vi "Dashboard Main.vi"() -> ()   [LabVIEW 2017]
uses:
  <vilib>/Utility/miscctls.llb/LVRowAndColumnTypeDef.ctl
  <vilib>/event_ctls.llb/eventvkey.ctl
  <vilib>/Rock Robotics/Network Tables/NT Read Numeric Array.vi
  <vilib>/Rock Robotics/Network Tables/NT Write Boolean.vi
  <vilib>/Rock Robotics/WPI/Dashboard/WPI_DashboardLogging Global.vi
panel:
  in  "TCP":refnum<k5>
  in  "Rec Mode":enum32{"Stop", "Record", "Playback"}(radio)
  out "Robot IP":string
  out "Image Message":string="Timeout in Camera Communications"
  in  "Dashboard Tab":T1(tab)
  in  "Drive Type":string(combo)
  in  "ResetGyro":bool
  in  "ResetSwerves":bool
  in  "Select Auto":string(combo)="Select Autonomous ..."
  out "NT Connection":bool
  out "MotorChart R":cluster{"Numeric":dbl, "Numeric":dbl}(graph)
  out "MotorChart L":cluster{"Numeric":dbl, "Numeric":dbl}(graph)
  out "MotorSliders R":cluster{"MotorSlide1":dbl, "MotorSlide2":dbl} {"MotorSlide2" scale=-1.0..1.0 scale format="%#_2e"; "MotorSlide1" scale=-1.0..1.0 scale format="%#_2e"}
  out "MotorSliders L":cluster{"MotorSlide1":dbl, "MotorSlide2":dbl} {"MotorSlide2" scale=-1.0..1.0 scale format="%#_2e"; "MotorSlide1" scale=-1.0..1.0 scale format="%#_2e"}
  out "Gyro":dbl(knob) scale=0.0..360.0
  out "JS1 Z":dbl(slide) scale=-1.0..1.0 scale format="%#_2e"
  out "JS1 Graph":cluster{"X":dbl, "Y":dbl}[](graph)
  out "JS1 Buttons":T2
  out "JS2 Z":dbl(slide) scale=-1.0..1.0 scale format="%#_2e"
  out "JS2 Graph":cluster{"X":dbl, "Y":dbl}[](graph)
  out "JS2 Buttons":T2
  out "Mode":T3(ring)=enum."Auto Disabled"
  in  "DB/String 9":string
  in  "DB/String 8":string
  in  "DB/String 7":string
  in  "DB/String 6":string
  in  "DB/String 5":string
  in  "DB/String 4":string
  in  "DB/String 3":string
  in  "DB/String 2":string
  in  "DB/String 1":string
  in  "DB/String 0":string
  in  "DB/Slider 0":dbl(slide) scale=0.0..5.0
  in  "DB/Slider 1":dbl(slide) scale=0.0..5.0
  in  "DB/Slider 2":dbl(slide) scale=0.0..5.0
  in  "DB/Slider 3":dbl(slide) scale=0.0..5.0
  out "DB/LED 3":bool
  out "DB/LED 2":bool
  out "DB/LED 1":bool
  out "DB/LED 0":bool
  in  "DB/Button 3":bool
  in  "DB/Button 2":bool
  in  "DB/Button 1":bool
  in  "DB/Button 0":bool caption="New Name"
  in  "Test Slider":dbl(slide) scale=0.0..100.0 scale format="%#_3g"
  in  "On/Off":bool caption="Solenoid"
  in  "Test Name":u16(ring) items=["Select the test to run..."]
  in  "Test Tree":string(tree)
  in  "Motor":cluster{"Value":dbl, "Enable":bool} {"Value" scale=-1.0..1.0 scale format="%#_3g"}
  out "Progress":T4 {"Test Progress" scale=0.0..100.0}
  in  "Rev/Fwd":cluster{"Forward":bool, "Reverse":bool}
  in  "Test Ring":u16(ring) items=["Monochrome", "Color"]
  out "Cmd Status":string
  in  "Execute Command":bool
  in  "Command Params":string[][](table)
  in  "Command Selection":i32(listbox)
  in  "CheckList":i32(listbox)
  out "Tree":string(tree)
  out "Background":bool
  # "Joysticks"
  # "Drive Motors"
  # "Front"
  # "Right"
  # "Left"
  # "Back"
  # "This tab is a great place for autonomous settings and robot-specific values.\nPlace controls and indicators inside this tab and match name to\nDashboard Variables on robot. You can also delete this comment."
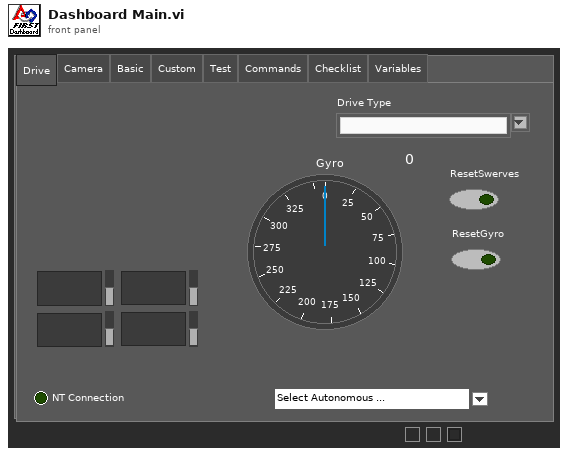
[diagram p1: front panel]
types:
  T1 = enum32{"Drive", "Camera", "Basic", "Custom", "Test", "Commands", "Checklist", "Variables"}
  T2 = cluster{bool, bool, bool, bool, bool, bool, bool, bool, bool, bool, bool, bool}
  T3 = enum8{"Tele-Op Disabled", "Tele-Op Enabled", "Auto Disabled", "Auto Enabled", "Test Disabled", "Test Enabled", "Disconnected", "No Code", "E-Stop"}
  T4 = cluster{"Test Progress":u8, "Test Progress Text":string}
  T5 = cluster{"IDs":cluster{"RPC field ID":u16, "Unique ID":u16}, "String":string}
  T6 = cluster{"Error Strings":string, "Disable Counts":cluster{u16, u16}, "Rail Faults":cluster{u16, u16, u16}, "Robot IP":string, "DB Mode":u8, "Event Info":cluster{"Name":string, "Type":u8, "Number":u16, "Replay":u8}}
  T7 = cluster{"Storage":cluster{"Disk Free":u64, "RAM Block":u32, "RAM free":u32}, "CPU Utilization":cluster{"CPU % ISR":sgl, "CPU % Time Crit":sgl, "CPU % Timed Str":sgl, "CPU % High":sgl, "CPU % Above":sgl, "CPU % Normal":sgl, "CPU % Low":sgl}, "CAN":cluster{"% Bus Utilization":sgl, "Bus Off Cnt":u32, "TX_FIFO Full Cnt":u32, "Receive Error Cnt":u8, "Transmit Error Cnt":u8}, "HID":cluster{"HID Outputs":u32, "Rumble Low":u16, "Rumble High":u16}[]}
  T8 = cluster{"Status bits":cluster{"Test Mode":bool, "Autonomous":bool, "Enabled":bool, "Code Start":bool, "Brownout":bool, "Reserved 2":bool, "Reserved 3":bool, "E-Stop":bool}, "Code Trace":cluster{"Disabled":bool, "TeleOp":bool, "Auto":bool, "Test":bool}, "Controller Type":enum16{"unknown", "cRIO", "roboRio"}, "Code?":enum16{"unknown", "noCode", "code"}, "Battery V":dbl}
  T9 = cluster{"Control Bits":cluster{"TestMode":bool, "Autonomous":bool, "Enabled":bool, "FMS Present":bool, bool, bool, bool, "E-Stop":bool}, "Team Station ":u8, "Countdown":sgl, "Joystick Values":cluster{"Axes":dbl[], "Buttons":bool[], "POVs":i16[]}[]}
  T10 = cluster{"Axes":dbl[], "Buttons":bool[], "POVs":i16[]}[]
  T11 = cluster{"Axes":dbl[], "Buttons":bool[], "POVs":i16[]}
  T12 = cluster{"Buttons[0]":bool, "Buttons[1]":bool, "Buttons[2]":bool, "Buttons[3]":bool, "Buttons[4]":bool, "Buttons[5]":bool, "Buttons[6]":bool, "Buttons[7]":bool, "Buttons[8]":bool, "Buttons[9]":bool, "Buttons[10]":bool, "Buttons[11]":bool}
  T13 = cluster{"Operation":enum16{"Update", "Clear"}, "Color Box":u32}[]
  T14 = typedef "eventvkey.ctl" = enum16{"ASCII", "Enter", "Return", "Shift", "Ctrl", "Alt", "Cmd", "Opt", "Caps", "NumLock", "Clear", "Break", "Up", "Down", "Left", "Right", "Insert", "Delete", "Home", "End", "PageUp", "PageDown", "Escape", "Help", "Pause", "ScrollLock", "F1", "F2", "F3", "F4", "F5", "F6", "F7", "F8", "F9", "F10", "F11", "F12", "F13", "F14", "F15", "F16", "F17", "F18", "F19", "F20", "F21", "F22", "F23", "F24", "Play", "VolumeUp", "VolumeDown", "Mute", "Two Byte Char"}
  T15 = cluster{"Image Size":bool, "Image Type":bool, "Pixel Value":bool, "ROI Information":bool, "Zoom Factor":bool}
  T16 = cluster{"Operation":enum16{"Update", "Clear"}, "Color Box":u32}
  T17 = typedef "LVRowAndColumnTypeDef.ctl" = cluster{"Row":i32, "Column":i32}
  T18 = cluster{"Shift":bool, "Ctrl":bool, "Alt":bool, "Cmd":bool, "Opt":bool}
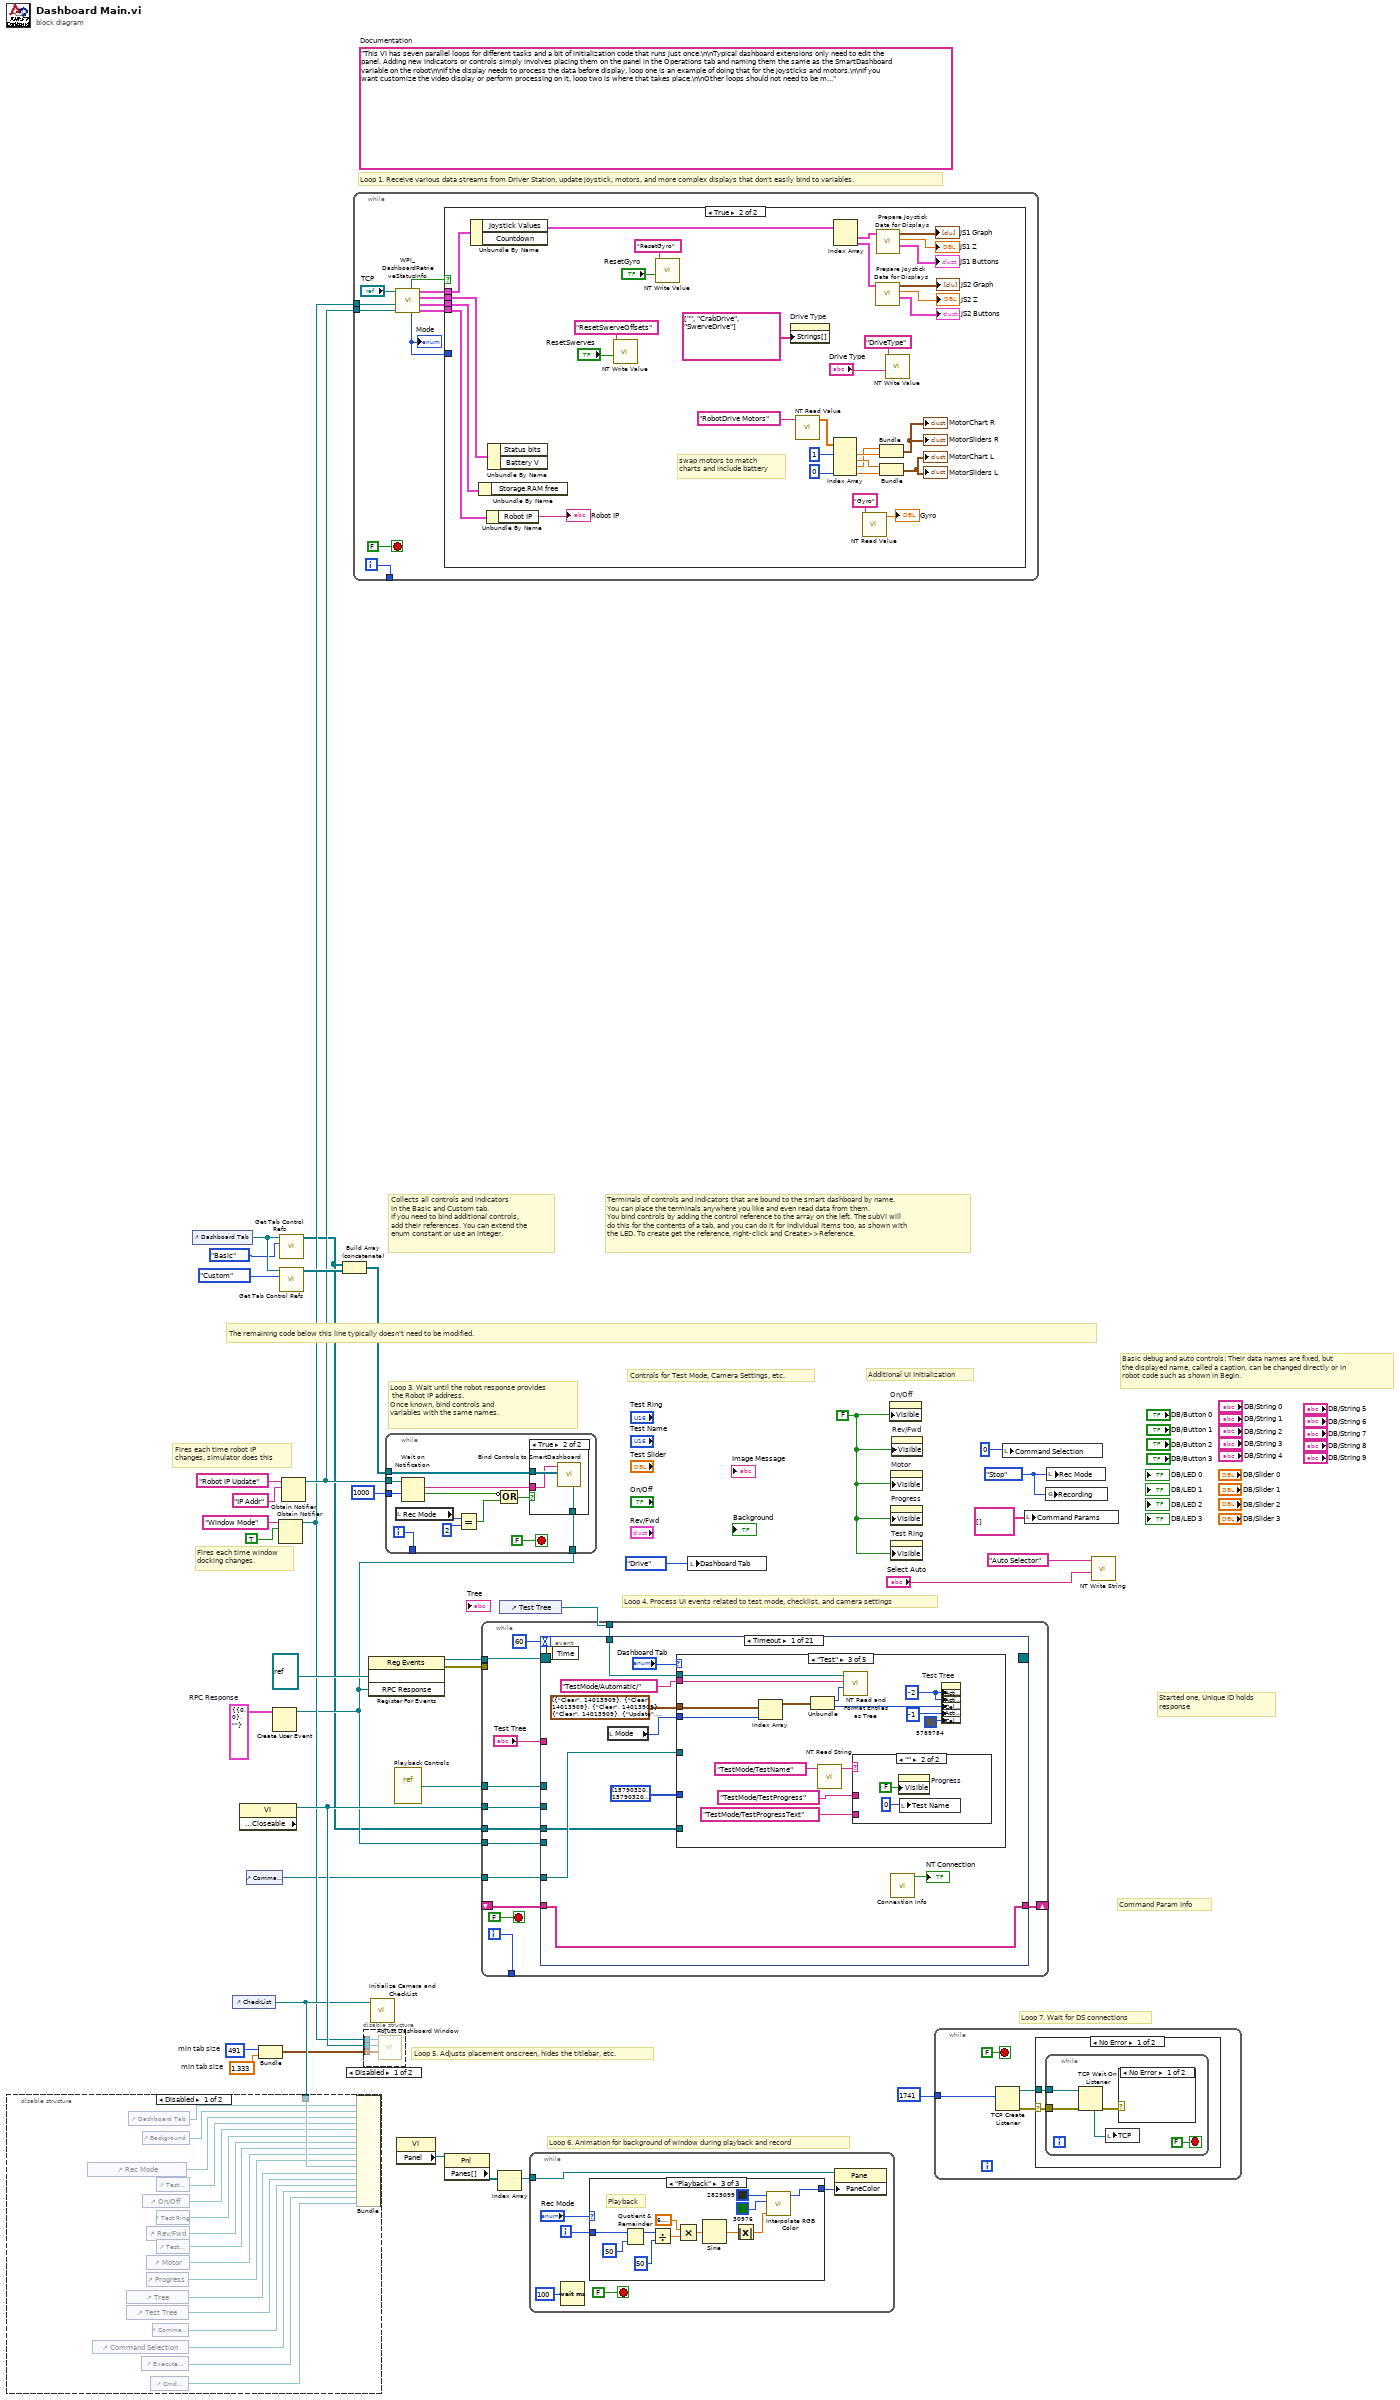
[diagram p0: block diagram]
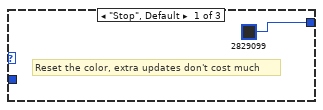
[diagram p4: hidden frame]
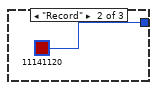
[diagram p5: hidden frame]
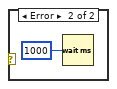
[diagram p6: hidden frame]
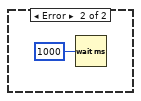
[diagram p7: hidden frame]
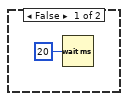
[diagram p8: hidden frame]
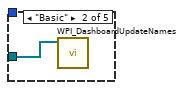
[diagram p11: hidden frame]
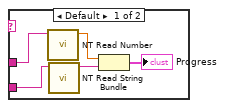
[diagram p12: hidden frame]
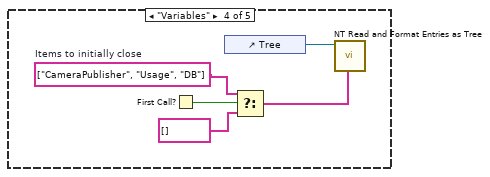
[diagram p13: hidden frame]
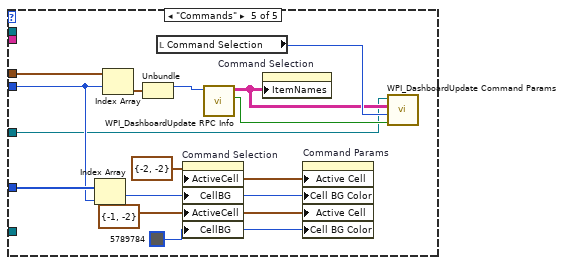
[diagram p14: hidden frame]
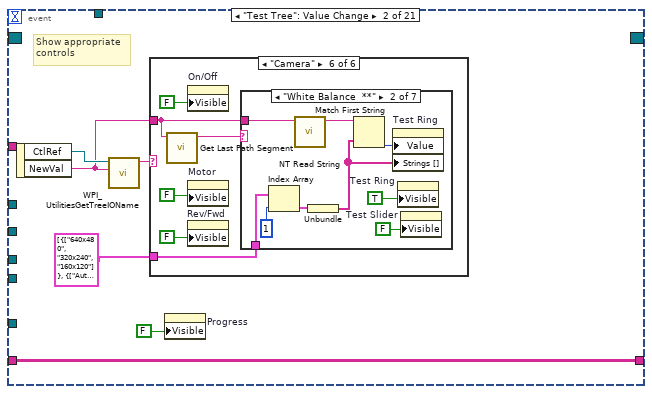
[diagram p15: hidden frame]
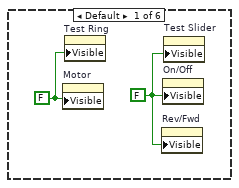
[diagram p16: hidden frame]
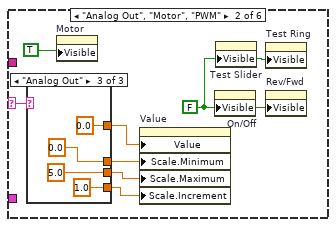
[diagram p17: hidden frame]
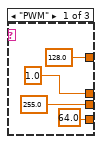
[diagram p18: hidden frame]
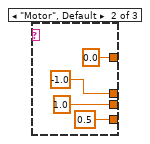
[diagram p19: hidden frame]
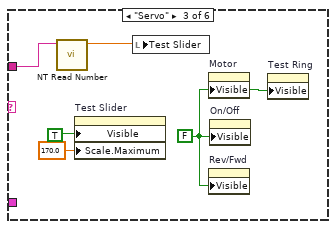
[diagram p20: hidden frame]
diagram:
  w3 = 491  # min tab size
  w2 = 1.333  # min tab size
  w16 = T5 {"IDs"={"RPC field ID"=0, "Unique ID"=0}, "String"=""}  # RPC Response
  w27 = enum32{"Stop", "Record", "Playback"}."Stop" ("Rec Mode")
  w21 = FALSE ("Visible")
  (unwired) "This VI has seven parallel loops for different tasks and a bit of initialization code that runs just once.\n\nTypical dashboard extensions only need to edit the panel. Adding new indicators or controls simply involves placing them on the panel in the Operations tab and naming them the same as the SmartDashboard variable on the robot\n\nIf the display needs to process the data before display, loop one is an example of doing that for the joysticks and motors.\n\nIf you want customize the video display or perform processing on it, loop two is where that takes place.\n\nOther loops should not need to be modified. They are pretty standard, and document the task they perform."  # Documentation
  # "Loop 5. Adjusts placement onscreen, hides the titlebar, etc."
  # "Loop 6. Animation for background of window during playback and record"
  # "Command Param Info"
  # "Started one, Unique ID holds\nresponse"
  # "Loop 7. Wait for DS connections"
  # "Basic debug and auto controls: Their data names are fixed, but\nthe displayed name, called a caption, can be changed directly or in\nrobot code such as shown in Begin."
  # "Controls for Test Mode, Camera Settings, etc."
  # "Additional UI Initialization"
  # "Fires each time robot IP\nchanges, simulator does this"
  # "Fires each time window\ndocking changes."
  # "Collects all controls and indicators\nin the Basic and Custom tab.\nIf you need to bind additional controls,\nadd their references. You can extend the\nenum constant or use an integer."
  # "The remaining code below this line typically doesn't need to be modified."
  # "Loop 4. Process UI events related to test mode, checklist, and camera settings"
  # "Terminals of controls and indicators that are bound to the smart dashboard by name.\nYou can place the terminals anywhere you like and even read data from them.\nYou bind controls by adding the control reference to the array on the left. The subVI will\ndo this for the contents of a tab, and you can do it for individual items too, as shown with\nthe LED. To create get the reference, right-click and Create>>Reference."
  # "Loop 3. Wait until the robot response provides\n the Robot IP address.\nOnce known, bind controls and\nvariables with the same names."
  # "Loop 1. Receive various data streams from Driver Station, update joystick, motors, and more complex displays that don't easily bind to variables."
  n1 = control-ref of="Dashboard Tab"() -> (w25:refnum<vi>)
  n2 = control-ref of="CheckList"() -> (w22:refnum<vi>)
  n3 = disable-structure shown="Disabled" {
    disable-tunnel: w22 -> [w54 _]
    frame Disabled {
      n4 = control-ref of="Rec Mode"() -> (w47:refnum<vi>)
      n5 = control-ref of="Command Selection"() -> (w39:refnum<vi>)
      n6 = control-ref of="Tree"() -> (w51:refnum<vi>)
      n7 = control-ref of="Test Tree"() -> (w50:refnum<vi>)
      n8 = control-ref of="Dashboard Tab"() -> (w53:refnum<vi>)
      n9 = control-ref of="Execute Command"() -> (w40:refnum<vi>)
      n10 = control-ref of="Background"() -> (w52:refnum<vi>)
      n11 = control-ref of="On/Off"() -> (w45:refnum<vi>)
      n12 = control-ref of="Progress"() -> (w42:refnum<vi>)
      n13 = control-ref of="Rev/Fwd"() -> (w43:refnum<vi>)
      n14 = control-ref of="Motor"() -> (w48:refnum<vi>)
      n15 = control-ref of="Cmd Status"() -> (w38:refnum<vi>)
      n16 = control-ref of="Command Params"() -> (w41:refnum<vi>)
      n17 = control-ref of="Test Slider"() -> (w46:refnum<vi>)
      n18 = control-ref of="Test Ring"() -> (w44:refnum<vi>)
      n19 = control-ref of="Test Name"() -> (w49:refnum<vi>)
      n20 = Bundle("Dashboard Tab"=w53, "Background"=w52, "Rec Mode"=w47, "Test Slider"=w46, "On/Off"=w45, "Test Ring"=w44, "Rev/Fwd"=w43, "Test Name"=w49, "Motor"=w48, "Progress"=w42, "CheckList"=w54, "Tree"=w51, "Test Tree"=w50, "Command Params"=w41, "Command Selection"=w39, "Execute Command"=w40, "Cmd Status"=w38) -> ()  [unwired: 2 in, 1 out]
    }
    frame Enabled {
    }
  }
  n21 = property class="VI" props=["Front Panel.Closeable"]() -> (reference out=w26:refnum<vi>)  [unwired: 2 in, 2 out]
  n22 = control-ref of="Command Params"() -> (w12:refnum<vi>)
  n23 = Bundle("min tab size"=w3, "min tab size"=w2) -> (w1:cluster{"min tab size":i32, "min tab size":dbl})  [unwired: 1 in]
  n24 = Create User Event(user event datatype=w16) -> (user event=w13:refnum<user-event>)  [unwired: 1 in, 1 out]
  n25 = Obtain Notifier(name (unnamed)="Window Mode", notification data type=TRUE) -> (notifier out=w19:refnum<notifier>)  [unwired: 2 in, 2 out]
  n26 = call <vilib>:"Get Tab Control Refs.vi"("Page Index"=T1."Basic" ("Dashboard Tab"), "TabControl in"=w25) -> ("ControlsOnPage"=w11:refnum<vi>[])  [unwired: 9 in]
  n27 = call <vilib>:"Get Tab Control Refs.vi"("Page Index"=T1."Custom" ("Dashboard Tab"), "TabControl in"=w25) -> ("ControlsOnPage"=w24:refnum<vi>[])  [unwired: 9 in]
  n28 = Obtain Notifier(name (unnamed)="Robot IP Update", notification data type="IP Addr" ("name (unnamed)")) -> (notifier out=w20:refnum<notifier>)  [unwired: 2 in, 2 out]
  n29 = Build Array (concatenate)(w11, w24) -> (w23:refnum<vi>[])
  n30 = while {
    tunnel: [w64] -> _
    tunnel: w20 -> [w58]
    tunnel: w19 -> [w55]
    i -> [w64]
    stop <- FALSE stop-if-true
    n31 = call <vilib>:"WPI_DashboardRetrieveStatusInfo.vi"("Binding Refnum"=w58, "Window Mode Notifier"=w55, "TCP Cnx"="TCP") -> ("Power and Errors"=w59:T6, "Robot Metrics"=w62:T7, "Status Info"=w63:T8, "Control Info"=w60:T9, "Robot Mode"=w57:T3, "Process?"=w61:bool)  [unwired: 3 in]
    "Mode" <- w57
    n32 = case shown="True" w61 {
      tunnel: w63 -> [_ w99]
      tunnel: w62 -> [_ w98]
      tunnel: w60 -> [_ w97]
      tunnel: w59 -> [_ w96]
      tunnel: w57 -> [_ _]
      frame False {
        n33 = Wait (ms)(milliseconds to wait=u32 20) -> ()  [unwired: 1 out]
      }
      frame True {
        # "swap motors to match\ncharts and include battery"
        n34 = Unbundle By Name(w97) -> ("Joystick Values"=w87:T10)  [unwired: 1 out]
        n35 = Unbundle By Name(w98) -> ()  [unwired: 1 out]
        n36 = Unbundle By Name(w96) -> ("Robot IP"=→"Robot IP":string)
        n37 = Unbundle By Name(w99) -> ()  [unwired: 2 out]
        n38 = call-poly <vilib>:"NT Write Value.vi"("Boolean"="ResetSwerves", "Name"="ResetSwerveOffsets") -> ()  [unwired: 9 in, 1 out]
        n39 = call-poly <vilib>:"NT Write Value.vi"("Boolean"="ResetGyro", "Name"="ResetGyro") -> ()  [unwired: 9 in, 1 out]
        n40 = property on="Drive Type" class="CmbBox"("Strings[]"=string[] ["", "CrabDrive", "SwerveDrive"] ("Strings []")) -> ()  [unwired: 2 in, 2 out]
        n41 = call-poly <vilib>:"NT Read Value.vi"("Name"="RobotDrive Motors") -> ("Numeric Array"=w77:dbl[])  [unwired: 9 in, 1 out]
        n42 = Index Array(array=w77, index #1=1, index #4=0) -> (element #1=w91:dbl, element #2=w92:dbl, element #3=w90:dbl, element #4=w95:dbl)  [unwired: 2 in]
        n43 = Index Array(array=w87) -> (element #1=w86:T11, element #2=w82:T11)  [unwired: 2 in]
        n44 = call-poly <vilib>:"NT Read Value.vi"("Name"="Gyro") -> ("Numeric"=→"Gyro":dbl)  [unwired: 9 in, 1 out]
        n45 = call "Prepare Joystick Data for Displays.vi"("Joystick Values"=w82) -> ("Buttons"=→"JS2 Buttons":T12, "Z Axis"=→"JS2 Z":dbl, "Cartesian Data"=→"JS2 Graph":cluster{"X axis":dbl, "X axis":dbl}[])  [unwired: 8 in]
        n46 = call "Prepare Joystick Data for Displays.vi"("Joystick Values"=w86) -> ("Buttons"=→"JS1 Buttons":T12, "Z Axis"=→"JS1 Z":dbl, "Cartesian Data"=→"JS1 Graph":cluster{"X axis":dbl, "X axis":dbl}[])  [unwired: 8 in]
        n47 = Bundle("Numeric"=w90, "Numeric"=w91) -> (→"MotorChart R" →"MotorSliders R":cluster{"Numeric":dbl, "Numeric":dbl})  [unwired: 1 in]
        n48 = Bundle("Numeric"=w92, "Numeric"=w95) -> (→"MotorChart L" →"MotorSliders L":cluster{"Numeric":dbl, "Numeric":dbl})  [unwired: 1 in]
        n49 = call-poly <vilib>:"NT Write Value.vi"("String"="Drive Type", "Name"="DriveType") -> ()  [unwired: 9 in, 1 out]
      }
    }
  }
  n50 = disable-structure shown="Disabled" {
    disable-tunnel: w26 -> [w102 _]
    disable-tunnel: w19 -> [w101 _]
    disable-tunnel: w1 -> [w100 _]
    frame Disabled {
      n51 = call "Adjust Dashboard Window.vi"("Size Constraints"=w100, "VI"=w102, "WIn Mode"=w101) -> ()  [unwired: 9 in]
    }
    frame Enabled {
    }
  }
  n52 = register-events(refnum<vi> refnum, w13) -> (reference out=w31:refnum<event-registration>, error out=w30:errorcluster)  [unwired: 2 in]
  n53 = call "Initialize Camera and CheckList.vi"("ListBox in"=w22) -> ()  [unwired: 11 in]
  n54 = while {
    tunnel: w23 -> [w114]
    tunnel: w20 -> [w112]
    tunnel: [w110] -> _
    tunnel: u32 1000 ("milliseconds to wait") -> [w109]
    tunnel: w13 -> [w103]
    i -> [w110]
    stop <- FALSE stop-if-true
    n55 = local read "Rec Mode"() -> (w105:enum32{"Stop", "Record", "Playback"})
    n56 = Wait on Notification(notifier=w112, timeout in ms (-1)=w109) -> (notification=w111:string, timed out?=w107:bool)  [unwired: 2 in, 2 out]
    n57 = Equal?(x=w105, y=u16 2 ("Rec Mode")) -> (x = y?=w106:bool)
    n58 = Compound Arithmetic op=OR(invert w107, w106) -> (w108:bool)
    n59 = case shown="True" w108 {
      tunnel: w114 -> [_ w117]
      tunnel: w111 -> [_ w116]
      tunnel: w103 -> [_ w115]
      frame False {
      }
      frame True {
        n60 = call <vilib>:"Bind Controls to SmartDashboard.vi"("RPC ref"=w115, "Bound Control Refs"=w117, "Server IP Address"=w116) -> ()  [unwired: 9 in]
      }
    }
  }
  n61 = vi-ref "Playback Controls.vi"() -> (w32:refnum<vi>)
  n62 = property class="VI"() -> ("Panel"=w5:refnum<vi>)  [unwired: 2 in, 2 out]
  n63 = property class="Pnl"(reference=w5) -> ("Panes[]"=w6:refnum<vi>[])  [unwired: 1 in, 2 out]
  n64 = Index Array(array=w6) -> (element=w4:refnum<vi>)  [unwired: 1 in]
  n65 = control-ref of="Test Tree"() -> (w33:refnum<vi>)
  n66 = while {
    tunnel: [w127] -> _
    tunnel: w33 -> [w126]
    tunnel: w32 -> [w125]
    tunnel: w31 -> [w124]
    tunnel: w30 -> [_]
    tunnel: w26 -> [w123]
    tunnel: w13 -> [w122]
    tunnel: w12 -> [w121]
    shift-right: [w120] -> _
    shift-left: _ -> [w119]
    tunnel: w11 -> [w118]
    i -> [w127]
    stop <- FALSE stop-if-true
    n67 = event shown="[0] Timeout" {
      selector: w124 -> [_ _ _ _ _ _ _ _ _ _ _ _ _ _ _ _ _ _ _ _ _]
      dyn-events: [_ _ _ _ _ _ _ _ _ _ _ _ _ _ _ _ w385 _ _ _ _] -> _
      timeout: u32 60 ("milliseconds to wait") -> [_ _ _ _ _ _ _ _ _ _ _ _ _ _ _ _ _ _ _ _ _]
      tunnel: w126 -> [w139 _ _ _ _ _ _ _ _ _ _ _ _ _ _ _ _ _ _ _ _]
      tunnel: "Test Tree" -> [_ _ _ _ _ _ _ _ _ _ _ w354 w362 w364 w368 w376 _ _ _ _ _]
      tunnel: w125 -> [_ _ _ _ _ _ _ _ _ _ _ _ _ _ _ _ w387 _ w405 _ _]
      tunnel: w123 -> [_ _ _ _ _ _ _ _ _ _ _ _ _ _ _ _ w383 _ _ _ _]
      tunnel: w122 -> [_ _ _ _ _ _ _ _ _ _ _ _ _ _ _ _ w381 _ _ _ _]
      tunnel: w121 -> [w134 _ _ _ _ _ w305 _ _ _ _ _ _ _ _ _ _ _ _ _ _]
      tunnel: [w133 w182 w284 w289 w298 w302 w303 w312 w322 w329 w341 w353 w360 w363 w367 w375 w380 w400 w402 w406 w419] -> w120
      tunnel: w119 -> [w133 w182 w284 w289 w298 w302 w303 _ _ w329 w341 w353 w360 w363 w367 w375 w380 w400 w402 w406 w419]
      tunnel: w118 -> [w131 _ _ _ _ _ _ _ _ _ _ _ _ _ _ _ _ _ _ _ _]
      event Timeout {
        n68 = event-data() -> ()  [unwired: 1 in, 1 out]
        n69 = local read "Mode"() -> (w136:T3)
        n70 = case shown="\"Test\"" "Dashboard Tab" {
          tunnel: w139 -> [_ _ w155 _ _]
          tunnel: "TestMode/Automatic/" ("Name Pattern") -> [_ _ w154 _ _]
          tunnel: T13 [{"Operation"=enum."Clear", "Color Box"=14013909}, {"Operation"=enum."Clear", "Color Box"=14013909}, {"Operation"=enum."Clear", "Color Box"=14013909}, {"Operation"=enum."Clear", "Color Box"=14013909}, {"Operation"=enum."Update", "Color Box"=14013909}, {"Operation"=enum."Update", "Color Box"=16777215}, {"Operation"=enum."Clear", "Color Box"=14013909}, {"Operation"=enum."Clear", "Color Box"=14013909}, {"Operation"=enum."Clear", "Color Box"=14013909}] -> [_ _ w147 _ w175]
          tunnel: w136 -> [_ _ w146 _ w174]
          tunnel: u32[] [15790320, 15790320, 15790320, 15790320, 16777215, 16777215, 15790320, 15790320, 15790320] -> [_ _ _ _ w180]
          tunnel: w134 -> [_ _ _ _ w168]
          tunnel: w131 -> [_ w141 _ _ _]
          frame "Custom", Default {
          }
          frame "Basic" {
            n71 = call <vilib>:"WPI_DashboardUpdateNames.vi"("Controls on Tab"=w141) -> ()  [unwired: 11 in]
          }
          frame "Test" {
            w153 = -2 ("Active Item:Row Number")
            n72 = Index Array(array=w147, index=w146) -> (element=w148:T16)
            n73 = Unbundle(w148) -> ("Operation"=w149:enum16{"Update", "Clear"}, "Color Box"=w150:u32)
            n74 = call <vilib>:"NT Read String.vi"("Name"="TestMode/TestName") -> ("String"=w144:string)  [unwired: 9 in, 1 out]
            n75 = call <vilib>:"NT Read and Format Entries as Tree.vi"("Operation"=w149, "Name Pattern"=w154, "Tree Refnum"=w155) -> ()  [unwired: 7 in, 2 out]
            n76 = case shown="\"\"" w144 {
              tunnel: "TestMode/TestProgress" ("Name") -> [w157 _]
              tunnel: "TestMode/TestProgressText" ("Name") -> [w156 _]
              frame Default {
                n77 = call <vilib>:"NT Read Number.vi"("Name"=w157) -> ("Numeric"=w158:dbl)  [unwired: 9 in, 1 out]
                n78 = call <vilib>:"NT Read String.vi"("Name"=w156) -> ("String"=w159:string)  [unwired: 9 in, 1 out]
                n79 = Bundle("Numeric"=w158, "String"=w159) -> (→"Progress":cluster{"Numeric":dbl, "String":string})  [unwired: 1 in]
              }
              frame "" {
                n80 = property on="Progress" class="Clust (strict)"("Visible"=FALSE) -> ()  [unwired: 2 in, 2 out]
                n81 = local write "Test Name"(u16 0) -> ()
              }
            }
            n82 = property on="Test Tree" class="Tree (strict)"("Active Item Row Number"=w153, "ActiveColNum"=w153, "CellBG"=w150, "Active Item Row Number"=-1 ("Active Item:Row Number"), "CellBG"=u32 5789784 ("Color Box")) -> ()  [unwired: 2 in, 2 out]
          }
          frame "Variables" {
            w165 = string[] ["CameraPublisher", "Usage", "DB"]  # Items to initially close
            n83 = First Call?() -> (First Call?: T/F=w166:bool)
            n84 = control-ref of="Tree"() -> (w167:refnum<vi>)
            n85 = Select(t=w165, s=w166, f=string[] []) -> (s? t:f=w163:string[])
            n86 = call <vilib>:"NT Read and Format Entries as Tree.vi"("Tags to  Close"=w163, "Tree Refnum"=w167) -> ()  [unwired: 8 in, 2 out]
          }
          frame "Commands" {
            w176 = u32 5789784 ("Color Box")
            w177 = T17 {"Row"=-1, "Column"=-2} ("Active Cell:Active Cell")
            w179 = T17 {"Row"=-2, "Column"=-2} ("Active Cell:Active Cell")
            n87 = Index Array(array=w180, index=w174) -> (element=w178:u32)
            n88 = Index Array(array=w175, index=w174) -> (element=w173:T16)
            n89 = Unbundle(w173) -> ("Operation"=w172:enum16{"Update", "Clear"})  [unwired: 1 out]
            n90 = local read "Command Selection"() -> (w171:i32)
            n91 = property on="Command Selection" class="MCListbox (strict)"("ActiveCell"=w179, "CellBG"=w178, "ActiveCell"=w177, "CellBG"=w176) -> ()  [unwired: 2 in, 2 out]
            n92 = call <vilib>:"WPI_DashboardUpdate RPC Info.vi"("Operation"=w172) -> ("update"=w170:bool, "commands"=w169:string[][])  [unwired: 9 in]
            n93 = property on="Command Selection" class="MCListbox (strict)"("ItemNames"=w169) -> ()  [unwired: 2 in, 2 out]
            n94 = property on="Command Params" class="Tbl (strict)"("Active Cell"=w179, "Cell BG Color"=w178, "Active Cell"=w177, "Cell BG Color"=w176) -> ()  [unwired: 2 in, 2 out]
            n95 = call <vilib>:"WPI_DashboardUpdate Command Params.vi"("Update"=w170, "NewVal"=w171, "Commands"=w169, "Param Tbl"=w168) -> ()  [unwired: 7 in, 1 out]
          }
        }
        n96 = call <vilib>:"Connextion Info.vi"() -> ("Connected"=→"NT Connection":bool)  [unwired: 10 in, 1 out]
      }
      event "Test Tree": Value Change {
        # "Show appropriate\ncontrols"
        n97 = event-data() -> ("CtlRef"=w185:refnum<vi>, "NewVal"=w183:string)  [unwired: 1 in]
        n98 = call <vilib>:"WPI_UtilitiesGetTreeIOName.vi"("NewVal"=w183, "TreeControl in"=w185) -> ("I/O Name"=w186:string)  [unwired: 9 in]
        n99 = case shown="\"Camera\"" w186 {
          selector: w186 -> [_ w193 _ w215 w224 _]
          tunnel: w183 -> [_ _ w212 w214 _ w231]
          tunnel: cluster{string[]}[] [{["640x480", "320x240", "160x120"]}, {["Auto", "Fixed indoor", "Fixed outdoor 1", "Fixed outdoor 2", "Fixed fluorescent 1", "Fixed fluorescent 2", "Hold current"]}, {["Auto", "Flicker-free 50 Hz", "Flicker-free 60 Hz", "Hold current"]}, {["None", "Prioritize frame rate", "Prioritize image quality"]}, {["Monochrome", "Color"]}] -> [_ _ _ _ _ w230]
          frame Default {
            w188 = FALSE ("Visible")
            w187 = FALSE ("Visible")
            n100 = property on="Motor" class="Clust (strict)"("Visible"=w187) -> ()  [unwired: 2 in, 2 out]
            n101 = property on="Test Ring" class="Ring (strict)"("Visible"=w187) -> ()  [unwired: 2 in, 2 out]
            n102 = property on="Rev/Fwd" class="Clust (strict)"("Visible"=w188) -> ()  [unwired: 2 in, 2 out]
            n103 = property on="On/Off" class="Bool (strict)"("Visible"=w188) -> ()  [unwired: 2 in, 2 out]
            n104 = property on="Test Slider" class="Slide (strict)"("Visible"=w188) -> ()  [unwired: 2 in, 2 out]
          }
          frame "Analog Out", "Motor", "PWM" {
            w194 = FALSE ("Visible")
            n105 = case shown="\"Analog Out\"" w193 {
              tunnel: [1.0 ("Value") -1.0 ("Value") 0.0 ("Value")] -> w192
              tunnel: [255.0 ("Value") 1.0 ("Value") 5.0 ("Value")] -> w191
              tunnel: [128.0 ("Value") 0.0 ("Value") 0.0 ("Value")] -> w190
              tunnel: [64.0 ("Value") 0.5 ("Value") 1.0 ("Value")] -> w189
              frame "PWM" {
              }
              frame "Motor", Default {
              }
              frame "Analog Out" {
              }
            }
            n106 = property on="Motor" class="Clust (strict)"("Visible"=TRUE) -> ()  [unwired: 2 in, 2 out]
            n107 = property on="Value" class="Slide (strict)"("Value"=w190, "Scale.Minimum"=w192, "Scale.Maximum"=w191, "Scale.Increment"=w189) -> ()  [unwired: 2 in, 2 out]
            n108 = property on="On/Off" class="Bool (strict)"("Visible"=w194) -> ()  [unwired: 2 in, 2 out]
            n109 = property on="Test Slider" class="Slide (strict)"("Visible"=w194) -> ()  [unwired: 2 in, 2 out]
            n110 = property on="Test Ring" class="Ring (strict)"("Visible"=w194) -> ()  [unwired: 2 in, 2 out]
            n111 = property on="Rev/Fwd" class="Clust (strict)"("Visible"=w194) -> ()  [unwired: 2 in, 2 out]
          }
          frame "Servo" {
            w210 = FALSE ("Visible")
            n112 = call <vilib>:"NT Read Number.vi"("Name"=w212) -> ("Numeric"=w211:dbl)  [unwired: 9 in, 1 out]
            n113 = property on="Test Slider" class="Slide (strict)"("Visible"=TRUE, "Scale.Maximum"=170.0 ("Scale.Range:Maximum")) -> ()  [unwired: 2 in, 2 out]
            n114 = local write "Test Slider"(w211) -> ()
            n115 = property on="Motor" class="Clust (strict)"("Visible"=w210) -> ()  [unwired: 2 in, 2 out]
            n116 = property on="Rev/Fwd" class="Clust (strict)"("Visible"=w210) -> ()  [unwired: 2 in, 2 out]
            n117 = property on="On/Off" class="Bool (strict)"("Visible"=w210) -> ()  [unwired: 2 in, 2 out]
            n118 = property on="Test Ring" class="Ring (strict)"("Visible"=w210) -> ()  [unwired: 2 in, 2 out]
          }
          frame "Relay", "Solenoid" {
            w213 = FALSE ("Visible")
            n119 = property on="Motor" class="Clust (strict)"("Visible"=w213) -> ()  [unwired: 2 in, 2 out]
            n120 = property on="Test Slider" class="Slide (strict)"("Visible"=w213) -> ()  [unwired: 2 in, 2 out]
            n121 = Search and Replace String(input string=w214, search string="/Value  **", replace string="/Direction") -> (result string=w220:string)  [unwired: 5 in, 3 out]
            n122 = property on="Test Ring" class="Ring (strict)"("Visible"=w213) -> ()  [unwired: 2 in, 2 out]
            n123 = call <vilib>:"NT Read String.vi"("Name"=w220) -> ("String"=w218:string)  [unwired: 9 in, 1 out]
            n124 = Equal?(x="Both directions", y=w218) -> (x = y?=w216:bool)
            n125 = Not(x=w216) -> (.not. x?=w217:bool)
            n126 = property on="Rev/Fwd" class="Clust (strict)"("Visible"=w216) -> ()  [unwired: 2 in, 2 out]
            n127 = property on="On/Off" class="Bool (strict)"("Visible"=w217, "Caption.Text"=w215) -> ()  [unwired: 2 in, 2 out]
          }
          frame "Compressor", "Digital Out" {
            w223 = FALSE ("Visible")
            # "Get direction and finish"
            n128 = property on="Motor" class="Clust (strict)"("Visible"=w223) -> ()  [unwired: 2 in, 2 out]
            n129 = property on="Test Slider" class="Slide (strict)"("Visible"=w223) -> ()  [unwired: 2 in, 2 out]
            n130 = property on="Test Ring" class="Ring (strict)"("Visible"=w223) -> ()  [unwired: 2 in, 2 out]
            n131 = property on="On/Off" class="Bool (strict)"("Visible"=TRUE, "Caption.Text"=w224) -> ()  [unwired: 2 in, 2 out]
            n132 = property on="Rev/Fwd" class="Clust (strict)"("Visible"=FALSE) -> ()  [unwired: 2 in, 2 out]
          }
          frame "Camera" {
            n133 = call <vilib>:"Get Last Path Segment.vi"("String in"=w231) -> ("String out"=w232:string)  [unwired: 10 in]
            n134 = property on="On/Off" class="Bool (strict)"("Visible"=FALSE) -> ()  [unwired: 2 in, 2 out]
            n135 = property on="Motor" class="Clust (strict)"("Visible"=FALSE) -> ()  [unwired: 2 in, 2 out]
            n136 = property on="Rev/Fwd" class="Clust (strict)"("Visible"=FALSE) -> ()  [unwired: 2 in, 2 out]
            n137 = case shown="\"White Balance  **\"" w232 {
              tunnel: w231 -> [w238 w247 w256 w265 w274 _ w280]
              tunnel: w230 -> [w236 w244 w253 w262 w271 _ _]
              frame "Size  **" {
                n138 = Index Array(array=w236) -> (element=w235:cluster{string[]})  [unwired: 1 in]
                n139 = call <vilib>:"NT Read String.vi"("Name"=w238) -> ("String"=w237:string)  [unwired: 9 in, 1 out]
                n140 = Unbundle(w235) -> (w233:string[])
                n141 = Match First String(2:w233, 3:w237) -> (0:w234:i32)  [unwired: 1 out]
                n142 = property on="Test Ring" class="Ring (strict)"("Value"=w234, "Strings []"=w233) -> ()  [unwired: 2 in, 2 out]
                n143 = property on="Test Ring" class="Ring (strict)"("Visible"=TRUE) -> ()  [unwired: 2 in, 2 out]
                n144 = property on="Test Slider" class="Slide (strict)"("Visible"=FALSE) -> ()  [unwired: 2 in, 2 out]
              }
              frame "White Balance  **" {
                n145 = Index Array(array=w244, index=1) -> (element=w245:cluster{string[]})
                n146 = call <vilib>:"NT Read String.vi"("Name"=w247) -> ("String"=w246:string)  [unwired: 9 in, 1 out]
                n147 = Unbundle(w245) -> (w242:string[])
                n148 = Match First String(2:w242, 3:w246) -> (0:w241:i32)  [unwired: 1 out]
                n149 = property on="Test Ring" class="Ring (strict)"("Value"=w241, "Strings []"=w242) -> ()  [unwired: 2 in, 2 out]
                n150 = property on="Test Ring" class="Ring (strict)"("Visible"=TRUE) -> ()  [unwired: 2 in, 2 out]
                n151 = property on="Test Slider" class="Slide (strict)"("Visible"=FALSE) -> ()  [unwired: 2 in, 2 out]
              }
              frame "Exposure  **" {
                n152 = Index Array(array=w253, index=2) -> (element=w254:cluster{string[]})
                n153 = call <vilib>:"NT Read String.vi"("Name"=w256) -> ("String"=w255:string)  [unwired: 9 in, 1 out]
                n154 = Unbundle(w254) -> (w250:string[])
                n155 = Match First String(2:w250, 3:w255) -> (0:w251:i32)  [unwired: 1 out]
                n156 = property on="Test Ring" class="Ring (strict)"("Value"=w251, "Strings []"=w250) -> ()  [unwired: 2 in, 2 out]
                n157 = property on="Test Ring" class="Ring (strict)"("Visible"=TRUE) -> ()  [unwired: 2 in, 2 out]
                n158 = property on="Test Slider" class="Slide (strict)"("Visible"=FALSE) -> ()  [unwired: 2 in, 2 out]
              }
              frame "Exposure Priority  **" {
                n159 = Index Array(array=w262, index=3) -> (element=w263:cluster{string[]})
                n160 = call <vilib>:"NT Read String.vi"("Name"=w265) -> ("String"=w264:string)  [unwired: 9 in, 1 out]
                n161 = Unbundle(w263) -> (w259:string[])
                n162 = Match First String(2:w259, 3:w264) -> (0:w260:i32)  [unwired: 1 out]
                n163 = property on="Test Ring" class="Ring (strict)"("Value"=w260, "Strings []"=w259) -> ()  [unwired: 2 in, 2 out]
                n164 = property on="Test Ring" class="Ring (strict)"("Visible"=TRUE) -> ()  [unwired: 2 in, 2 out]
                n165 = property on="Test Slider" class="Slide (strict)"("Visible"=FALSE) -> ()  [unwired: 2 in, 2 out]
              }
              frame "Color Enable  **" {
                n166 = Index Array(array=w271, index=4) -> (element=w272:cluster{string[]})
                n167 = call <vilib>:"NT Read String.vi"("Name"=w274) -> ("String"=w273:string)  [unwired: 9 in, 1 out]
                n168 = Unbundle(w272) -> (w268:string[])
                n169 = Match First String(2:w268, 3:w273) -> (0:w269:i32)  [unwired: 1 out]
                n170 = property on="Test Ring" class="Ring (strict)"("Value"=w269, "Strings []"=w268) -> ()  [unwired: 2 in, 2 out]
                n171 = property on="Test Ring" class="Ring (strict)"("Visible"=TRUE) -> ()  [unwired: 2 in, 2 out]
                n172 = property on="Test Slider" class="Slide (strict)"("Visible"=FALSE) -> ()  [unwired: 2 in, 2 out]
              }
              frame Default {
                n173 = property on="Test Ring" class="Ring (strict)"("Visible"=FALSE) -> ()  [unwired: 2 in, 2 out]
                n174 = property on="Test Slider" class="Slide (strict)"("Visible"=FALSE) -> ()  [unwired: 2 in, 2 out]
              }
              frame "Brightness  **", "Color Level  **", "Compression  **", "FPS  **", "Sharpness  **" {
                n175 = call <vilib>:"NT Read Number.vi"("Name"=w280) -> ("Numeric"=w279:dbl)  [unwired: 9 in, 1 out]
                n176 = local write "Test Slider"(w279) -> ()
                n177 = property on="Test Slider" class="Slide (strict)"("Visible"=TRUE, "Scale.Maximum"=100.0 ("Scale.Range:Maximum")) -> ()  [unwired: 2 in, 2 out]
                n178 = property on="Test Ring" class="Ring (strict)"("Visible"=FALSE) -> ()  [unwired: 2 in, 2 out]
              }
            }
          }
        }
        n179 = property on="Progress" class="Clust (strict)"("Visible"=FALSE) -> ()  [unwired: 2 in, 2 out]
      }
      event "Test Name": Mouse Enter {
        # "Populate the ring with the list of tests"
        n180 = event-data() -> ()  [unwired: 1 in, 1 out]
        n181 = call <vilib>:"NT Read String Array.vi"("Name"="TestMode/TestList") -> ("String Array"=w288:string[])  [unwired: 9 in, 1 out]
        n182 = Build Array (concatenate)("Select the test to run...", w288) -> (w287:string[])
        n183 = property on="Test Name" class="Ring (strict)"("Strings []"=w287) -> ()  [unwired: 2 in, 2 out]
      }
      event "Test Name": Value Change {
        w290 = FALSE ("Visible")
        # "Tell the robot the test name to run"
        n184 = event-data() -> ("NewVal"=w294:u16)  [unwired: 1 in]
        n185 = property on="Test Name" class="Ring (strict)"() -> ("Strings []"=w295:string[])  [unwired: 2 in, 2 out]
        n186 = local write "Progress"(T4 {"Test Progress"=0, "Test Progress Text"=""} ("Progress")) -> ()
        n187 = Index Array(array=w295, index=w294) -> (element=w293:string)
        n188 = call <vilib>:"NT Write String.vi"("String"=w293, "Name"="TestMode/TestName") -> ()  [unwired: 9 in, 1 out]
        n189 = property on="Progress" class="Clust (strict)"("Visible"=TRUE) -> ()  [unwired: 2 in, 2 out]
        n190 = property on="Motor" class="Clust (strict)"("Visible"=w290) -> ()  [unwired: 2 in, 2 out]
        n191 = property on="Test Slider" class="Slide (strict)"("Visible"=w290) -> ()  [unwired: 2 in, 2 out]
        n192 = property on="On/Off" class="Bool (strict)"("Visible"=w290) -> ()  [unwired: 2 in, 2 out]
        n193 = property on="Rev/Fwd" class="Clust (strict)"("Visible"=w290) -> ()  [unwired: 2 in, 2 out]
        n194 = property on="Test Ring" class="Ring (strict)"("Visible"=w290) -> ()  [unwired: 2 in, 2 out]
      }
      event "Select Auto": Mouse Enter {
        # "Populate the combo box with the list of autonomous options"
        n195 = event-data() -> ()  [unwired: 1 in, 1 out]
        n196 = call <vilib>:"NT Read String Array.vi"("Name"="Auto List") -> ("String Array"=w297:string[])  [unwired: 9 in, 1 out]
        n197 = property on="Select Auto" class="CmbBox"("Strings[]"=w297) -> ()  [unwired: 2 in, 2 out]
      }
      event "Select Auto": Value Change {
        # "User modified the Auto Selection. Write to NT variable so robot knows."
        n198 = event-data() -> ("NewVal"=w300:string)  [unwired: 1 in]
        n199 = call <vilib>:"NT Write String.vi"("String"=w300, "Name"="Auto Selector") -> ()  [unwired: 9 in, 1 out]
      }
      event "Command Selection": Value Change {
        # "Get the params and show in table"
        n200 = event-data() -> ("NewVal"=w306:i32)  [unwired: 1 in]
        n201 = property on="Command Selection" class="MCListbox (strict)"() -> ("ItemNames"=w304:string[][])  [unwired: 2 in, 2 out]
        n202 = call <vilib>:"WPI_DashboardUpdate Command Params.vi"("NewVal"=w306, "Commands"=w304, "Param Tbl"=w305) -> ()  [unwired: 8 in, 1 out]
      }
      event "Execute Command": Value Change {
        # "Started one, Unique ID holds\nresponse"
        n203 = event-data() -> ()  [unwired: 1 in, 1 out]
        n204 = property on="Command Selection" class="MCListbox (strict)"() -> ("ItemNames"=w317:string[][])  [unwired: 2 in, 2 out]
        n205 = Index Array(array=w317, index (row)="Command Selection", index (col)=0) -> (element=w315:string)
        n206 = call <vilib>:"Invoke Commands.vi"("Command Params"="Command Params", "Function Name"=w315) -> ("Params"=w311:u8, "Started"=w310:bool)  [unwired: 7 in, 1 out]
        n207 = Array Subset(array="Command Params", length (row)=w311) -> (w312:string[][])  [unwired: 3 in]
        n208 = Select(t="Executing" ("Cmd Status"), s=w310, f="" ("Cmd Status")) -> (s? t:f=→"Cmd Status":string)
      }
      event "Command Selection": Double Click {
        n209 = event-data() -> ("Row"=w325:i32)  [unwired: 1 in]
        n210 = property on="Command Selection" class="MCListbox (strict)"() -> ("ItemNames"=w328:string[][])  [unwired: 2 in, 2 out]
        n211 = local read "Command Params"() -> (w324:string[][])
        n212 = Index Array(array=w328, index (row)=w325, index (col)=0) -> (element=w326:string)
        n213 = call <vilib>:"Invoke Commands.vi"("Command Params"=w324, "Function Name"=w326) -> ("Params"=w323:u8, "Started"=w318:bool)  [unwired: 7 in, 1 out]
        n214 = Array Subset(array=w324, length (row)=w323) -> (w322:string[][])  [unwired: 3 in]
        n215 = Select(t="Executing" ("Cmd Status"), s=w318, f="" ("Cmd Status")) -> (s? t:f=w319:string)
        n216 = local write "Cmd Status"(w319) -> ()
      }
      event "CheckList": Double Click {
        # "Shift clears all"
        # "Update symbols on the listbox"
        n217 = event-data() -> ("PlatMods.Shift"=w330:bool, "Row"=w332:i32)  [unwired: 1 in]
        n218 = case shown="True" w330 {
          tunnel: w332 -> [w336 _]
          tunnel: 1 -> [w335 _]
          frame False {
            n219 = property on="CheckList" class="LstBox (strict)"() -> ("Item Symbols"=w334:i32[])  [unwired: 2 in, 2 out]
            n220 = Replace Array Subset(array=w334, new element=w335, index=w336) -> (w333:i32[])
            n221 = property on="CheckList" class="LstBox (strict)"("Item Symbols"=w333) -> ()  [unwired: 2 in, 2 out]
          }
          frame True {
            w337 = 0 ("Top Row")
            n222 = property on="CheckList" class="LstBox (strict)"() -> ("Number of Rows"=w339:u32)  [unwired: 2 in, 2 out]
            n223 = Initialize Array(0, w339) -> (w338:i32[])
            n224 = property on="CheckList" class="LstBox (strict)"("Top Row"=w337, "Value"=w337, "Item Symbols"=w338) -> ()  [unwired: 2 in, 2 out]
          }
        }
      }
      event "CheckList": Key Down {
        # "Update symbols on the listbox\nLeft and right keys check and uncheck"
        n225 = event-data() -> ("VKey"=w343:T14)  [unwired: 1 in]
        n226 = case shown="\"Left\", \"Right\"" w343 {
          selector: w343 -> [w348 _]
          tunnel: eventvkey."Left" ("VKey") -> [w346 _]
          frame "Left", "Right" {
            n227 = Equal?(x=w346, y=w348) -> (x = y?=w347:bool)
            n228 = Select(t=0, s=w347, f=1) -> (s? t:f=w349:i32)
            n229 = property on="CheckList" class="LstBox (strict)"() -> ("Item Symbols"=w352:i32[])  [unwired: 2 in, 2 out]
            n230 = Replace Array Subset(array=w352, new element=w349, index="CheckList") -> (w351:i32[])
            n231 = property on="CheckList" class="LstBox (strict)"("Item Symbols"=w351) -> ()  [unwired: 2 in, 2 out]
          }
          frame Default {
          }
        }
      }
      event "Motor.Enable": Value Change {
        # "When the test mode otor enable helper is set, update that\ntree row item's value"
        n232 = event-data() -> ("NewVal"=w358:bool)  [unwired: 1 in]
        n233 = Unbundle("Motor") -> ("Value"=w357:dbl)  [unwired: 1 out]
        n234 = Select(t=w357, s=w358, f=0.0) -> (s? t:f=w355:dbl)
        n235 = call <vilib>:"NT Write Number.vi"("Numeric"=w355, "Name"=w354) -> ()  [unwired: 9 in, 1 out]
      }
      event "Test Slider": Value Change {
        # "When the test mode slider helper is set, update that\ntree row item's value"
        n236 = event-data() -> ("NewVal"=w361:dbl)  [unwired: 1 in]
        n237 = call <vilib>:"NT Write Number.vi"("Numeric"=w361, "Name"=w362) -> ()  [unwired: 9 in, 1 out]
      }
      event "On/Off": Value Change {
        # "When the test mode on/off helper value is set, update that\ntree row item's value"
        n238 = event-data() -> ("NewVal"=w366:bool)  [unwired: 1 in]
        n239 = Boolean To (0,1)(Boolean=w366) -> (0, 1=w365:i16)
        n240 = call <vilib>:"NT Write Number.vi"("Numeric"=w365, "Name"=w364) -> ()  [unwired: 9 in, 1 out]
      }
      event "Rev/Fwd": Value Change {
        # "When the test mode helper value for relays is set, update that\ntree row item's value"
        n241 = event-data() -> ("NewVal.Forward"=w374:bool, "NewVal.Reverse"=w373:bool)  [unwired: 1 in]
        n242 = Boolean To (0,1)(Boolean=w374) -> (0, 1=w370:i16)
        n243 = Boolean To (0,1)(Boolean=w373) -> (0, 1=w372:i16)
        n244 = Negate(x=w372) -> (-x=w371:i16)
        n245 = Add(x=w370, y=w371) -> (x+y=w369:i16)
        n246 = call <vilib>:"NT Write Number.vi"("Numeric"=w369, "Name"=w368) -> ()  [unwired: 9 in, 1 out]
      }
      event "Test Ring": Value Change {
        # "When a test mode helper value is selected from the ring,\nset the tree item's variable to the string value"
        n247 = event-data() -> ("NewVal"=w378:u16)  [unwired: 1 in]
        n248 = property on="Test Ring" class="Ring (strict)"() -> ("Strings []"=w379:string[])  [unwired: 2 in, 2 out]
        n249 = Index Array(array=w379, index=w378) -> (element=w377:string)
        n250 = call <vilib>:"NT Write String.vi"("String"=w377, "Name"=w376) -> ()  [unwired: 9 in, 1 out]
      }
      event "Rec Mode": Value Change {
        # "Update globals for recording mode and path to read log from.\nClear when logging and let NetworkTables set path for vision to\nuse."
        n251 = event-data() -> ("NewVal"=w388:enum32{"Stop", "Record", "Playback"})  [unwired: 1 in]
        n252 = global write "WPI_DashboardLogging Global.vi" "Logging Filename"(path "") -> ()
        n253 = global write "WPI_DashboardLogging Global.vi" "Recording"(w388) -> ()
        n254 = case shown="\"Playback\"" w388 {
          tunnel: w387 -> [_ w390 w399]
          tunnel: [_ _ w398] -> w385
          tunnel: [_ _ w397] -> _
          tunnel: w383 -> [_ _ w395]
          tunnel: cluster{i32, i32} {-250, 170} -> [_ _ w394]
          tunnel: [_ _ T15 {"Image Size"=TRUE, "Image Type"=TRUE, "Pixel Value"=TRUE, "ROI Information"=TRUE, "Zoom Factor"=FALSE} ("Image Information Shown:All Elements")] -> _
          tunnel: [_ _ TRUE ("Zoom Factor")] -> _
          tunnel: w381 -> [_ _ w391]
          frame Default {
          }
          frame "Stop", "Record" {
            # "Place Window too"
            n255 = invoke class="VI" method="FP.Close"(reference=w390) -> (reference out=w389:refnum<vi>)  [unwired: 2 in, 2 out]
            n256 = invoke class="VI" method="Abort VI"(reference=w389) -> ()  [unwired: 2 in, 3 out]
          }
          frame "Playback" {
            n257 = call "Open Playback Panel.vi"("Offset"=w394, "DB VI Ref"=w395, "Playback in"=w399) -> ("Playback out"=w396:refnum<vi>)  [unwired: 8 in]
            n258 = register-events(w396, w391) -> (reference out=w398:refnum<event-registration>, error out=w397:errorcluster)  [unwired: 2 in]
          }
        }
        n259 = call <vilib>:"WPI_DashboardNT Log FieldName Cache.vi"("Operation"=enum16{"Lookup/Add", "Index", "Clear"}."Clear") -> ()  [unwired: 8 in, 3 out]
      }
      event Panel Close {
        w401 = enum32{"Stop", "Record", "Playback"}."Stop" ("Rec Mode")
        # "Playback window has been closed, abort"
        n260 = event-data() -> ()  [unwired: 1 in, 4 out]
        n261 = local write "Rec Mode"(w401) -> ()
        n262 = global write "WPI_DashboardLogging Global.vi" "Recording"(w401) -> ()
      }
      event Panel Close {
        # "Abort playback window and ourself"
        n263 = event-data() -> ()  [unwired: 1 in, 4 out]
        n264 = invoke class="VI" method="FP.Close"(reference=w405) -> (reference out=w404:refnum<vi>)  [unwired: 2 in, 2 out]
        n265 = invoke class="VI" method="Abort VI"(reference=w404) -> (error out=w403:errorcluster)  [unwired: 2 in, 2 out]
        n266 = invoke class="VI" method="Abort VI"(error in=w403) -> ()  [unwired: 2 in, 3 out]
      }
      event User Event {
        n267 = event-data() -> ("IDs"=w412:cluster{"RPC field ID":u16, "Unique ID":u16}, "String"=w411:string)  [unwired: 1 in]
        n268 = Bundle("IDs"=w412, "String"=w411) -> (w410:T5)  [unwired: 1 in]
        n269 = call <vilib>:"Retrieve RPC Response.vi"("RPC Response"=w410) -> ("Output"=w408:string[][])  [unwired: 10 in]
        n270 = Build Array (concatenate)(w406, w408) -> (w407:string[][])
        n271 = local write "Command Params"(w407) -> ()
        n272 = local write "Cmd Status"("" ("Cmd Status")) -> ()
      }
      event "Tree": Double Click {
        n273 = event-data() -> ("PlatMods"=w418:T18, "Tag"=w415:string)  [unwired: 1 in]
        n274 = Unbundle(w418) -> ("Shift"=w417:bool)  [unwired: 4 out]
        n275 = String Subset(string=w415, length (rest)=1 ("length (rest)")) -> (substring=w414:string)  [unwired: 1 in]
        n276 = Not(x=w417) -> (.not. x?=w416:bool)
        n277 = case shown="\"/\"" w414 {
          tunnel: w415 -> [_ w421]
          tunnel: w416 -> [_ w420]
          frame Default {
          }
          frame "/" {
            n278 = call <vilib>:"NT Update Persistence.vi"("Persistence"=w420, "Name"=w421) -> ()  [unwired: 9 in, 1 out]
          }
        }
      }
    }
  }
  n279 = while {
    tunnel: w4 -> [w423]
    i -> [w426]
    stop <- FALSE stop-if-true
    n280 = Wait (ms)(milliseconds to wait=u32 100) -> ()  [unwired: 1 out]
    n281 = case shown="\"Playback\"" "Rec Mode" {
      tunnel: w426 -> [_ _ w441]
      tunnel: [u32 2829099 ("Base Color") u32 11141120 ("Target Color") w430] -> w422
      frame "Stop", Default {
        # "Reset the color, extra updates don't cost much"
      }
      frame "Record" {
      }
      frame "Playback" {
        # "Playback"
        n282 = Quotient & Remainder(x=w441, y=u32 50 ("milliseconds to wait")) -> (x-y*floor(x/y)=w437:u32)  [unwired: 1 out]
        n283 = Divide(x=w437, y=u32 50 ("milliseconds to wait")) -> (x/y=w434:dbl)
        n284 = Multiply(x=6.283185307179586, y=w434) -> (x*y=w439:dbl)
        n285 = Sine(x=w439) -> (sin(x)=w438:dbl)
        n286 = Absolute Value(x=w438) -> (abs(x)=w431:dbl)
        n287 = call "Interpolate RGB Color.vi"("Proportion"=w431, "Target Color"=u32 30976, "Base Color"=u32 2829099) -> ("Result Color"=w430:u32)  [unwired: 8 in]
      }
    }
    n288 = property class="Pane"(reference=w423, "PaneColor"=w422) -> ()  [unwired: 1 in, 2 out]
  }
  n289 = local write "Dashboard Tab"(T1."Drive" ("Dashboard Tab")) -> ()
  n290 = property on="On/Off" class="Bool (strict)"("Visible"=w21) -> ()  [unwired: 2 in, 2 out]
  n291 = property on="Motor" class="Clust (strict)"("Visible"=w21) -> ()  [unwired: 2 in, 2 out]
  n292 = property on="Progress" class="Clust (strict)"("Visible"=w21) -> ()  [unwired: 2 in, 2 out]
  n293 = property on="Test Ring" class="Ring (strict)"("Visible"=w21) -> ()  [unwired: 2 in, 2 out]
  n294 = property on="Rev/Fwd" class="Clust (strict)"("Visible"=w21) -> ()  [unwired: 2 in, 2 out]
  n295 = while {
    tunnel: u16 1741 ("timeout ms (25000)") -> [w443]
    stop <- FALSE stop-if-true
    n296 = TCP Create Listener(10:w443) -> (0:w442:errorcluster, 3:w444:refnum<k5>)  [unwired: 4 in, 1 out]
    n297 = case shown="No Error" w442 {
      selector: w442 -> [w446 _]
      tunnel: w444 -> [w447 _]
      frame No Error {
        n298 = while {
          tunnel: w447 -> [w450]
          tunnel: w446 -> [w449]
          stop <- FALSE stop-if-true
          n299 = TCP Wait On Listener(8:w449, 11:w450) -> (0:w451:errorcluster, 4:w452:refnum<k5>)  [unwired: 2 in, 3 out]
          n300 = local write "TCP"(w452) -> ()
          n301 = case shown="No Error" w451 {
            frame No Error {
            }
            frame Error {
              n302 = Wait (ms)(milliseconds to wait=u32 1000) -> ()  [unwired: 1 out]
            }
          }
        }
      }
      frame Error {
        n303 = Wait (ms)(milliseconds to wait=u32 1000) -> ()  [unwired: 1 out]
      }
    }
  }
  n304 = local write "Command Selection"(u16 0 ("milliseconds to wait")) -> ()
  n305 = local write "Command Params"(string[][] [] ("Command Params")) -> ()
  n306 = global write "WPI_DashboardLogging Global.vi" "Recording"(w27) -> ()
  n307 = local write "Rec Mode"(w27) -> ()
  n308 = call <vilib>:"NT Write String.vi"("String"="Select Auto", "Name"="Auto Selector") -> ()  [unwired: 9 in, 1 out]
